vi "Abstract method error.vi"(8 "error in (no error)":errorcluster) -> (0 "error out":errorcluster)   [LabVIEW 2016, in "RT Management.lvlib"]
uses:
  RT Management.lvlib
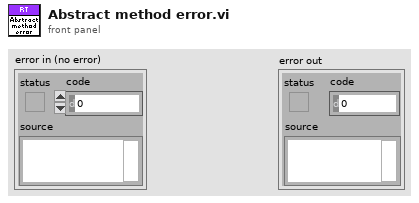
[diagram p1: front panel]
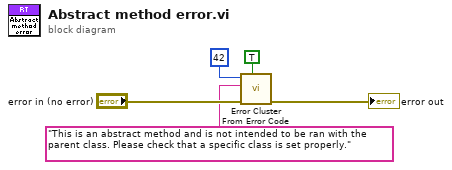
[diagram p0: block diagram]
diagram:
  n1 = call <vilib>:"Error Cluster From Error Code.vi"("show call chain? (False)"=TRUE, "error in (no error)"="error in (no error)", "error message (\"\")"="This is an abstract method and is not intended to be ran with the parent class. Please check that a specific class is set properly." ("error message (\"\")"), "error code (0)"=42) -> ("error out"=→"error out":errorcluster)  [unwired: 5 in]
